vi "Export - Rx Packets.vi"(8 "error in (no error)":errorcluster, 11 "Device Item Ref in":T5 format="%.0x") -> (0 "error out":errorcluster, 3 "Rx Packets":T1 {"Rx Packet Data"."Endianness" items=["big-endian"=0, "little-endian"=2]})   [LabVIEW 2016, in "UDP-Custom-Device System Explorer.lvlib"]
uses:
  UDP-Custom-Device System Explorer.lvlib
  <vilib>/NI Veristand/Custom Device API/Custom Device Item Ref.ctl
  Types/XML - New/ImpExp - Rx Packets Data.ctl
  <vilib>/NI Veristand/Custom Device API/Custom Device Item Info.ctl
  Types/XML - New/ImpExp - Rx Packet Data.ctl
  Shared/Types/Shared - Channel Data Type.ctl
  <vilib>/NI VeriStand/Custom Device API/Custom Device API.lvlib
  Property Accessors/Shared Section Accessors.lvlib
  Shared/UDP-Custom-Device Shared.lvlib
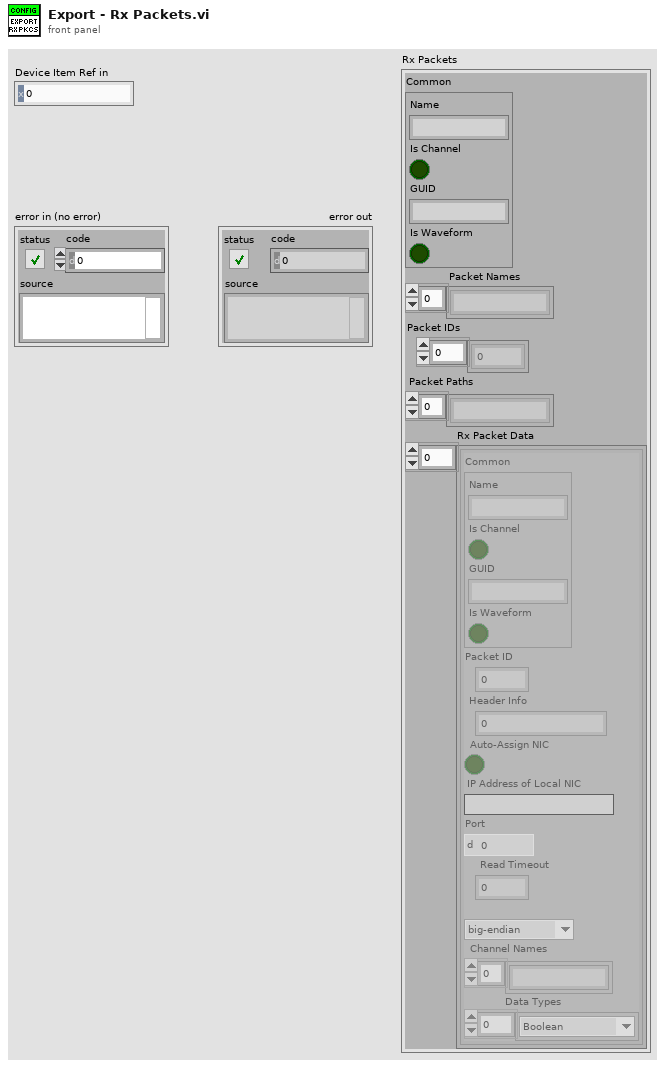
[diagram p1: front panel]
types:
  T1 = typedef "UDP-Custom-Device System Explorer.lvlib/ImpExp - Rx Packets Data.ctl" = cluster{"Common":T2, "Packet Names":string[], "Packet IDs":i32[], "Packet Paths":string[], "Rx Packet Data":T3[]}
  T2 = typedef "Custom Device API.lvlib/Custom Device Item Info.ctl" = cluster{"Name":string, "Is Channel":bool, "GUID":string, "Is Waveform":bool}
  T3 = typedef "UDP-Custom-Device System Explorer.lvlib/ImpExp - Rx Packet Data.ctl" = cluster{"Common":T2, "Packet ID":i32, "Header Info":u32, "Auto-Assign NIC":bool, "IP Address of Local NIC":string, "Port":u16, "Read Timeout":i32, "Endianness":u16, "Channel Names":string[], "Data Types":T4[]}
  T4 = typedef "UDP-Custom-Device Shared.lvlib/Shared - Channel Data Type.ctl" = enum16{"Boolean", "Single", "Double", "I8", "I16", "I32", "I64", "U8", "U16", "U32", "U64"}
  T5 = typedef "Custom Device API.lvlib/Custom Device Item Ref.ctl" = u64
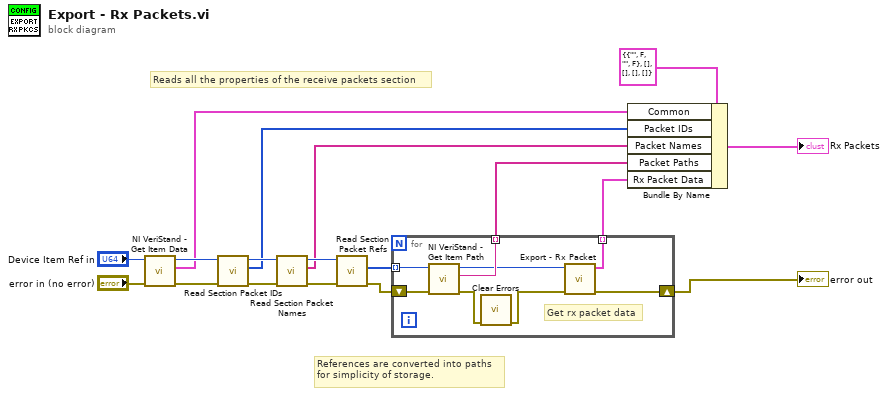
[diagram p0: block diagram]
diagram:
  # "References are converted into paths\nfor simplicity of storage."
  # "Reads all the properties of the receive packets section"
  n1 = call <vilib>:"NI VeriStand - Get Item Data.vi"("error in (no error)"="error in (no error)", "Item Ref in"="Device Item Ref in") -> ("error out"=w13:errorcluster, "Item Info"=w6:T2, "Item Ref out"=w18:T5)  [unwired: 6 in, 1 out]
  n2 = call "Read Section Packet IDs.vi"("error in (no error)"=w13, "Node Ptr"=w18) -> ("error out"=w15:errorcluster, "Packet IDs"=w5:i32[], "Node Ptr out"=w17:T5)  [unwired: 7 in]
  n3 = call "Read Section Packet Names.vi"("error in (no error)"=w15, "Node Ptr"=w17) -> ("error out"=w14:errorcluster, "Packet Names"=w4:string[], "Node Ptr out"=w16:T5)  [unwired: 7 in]
  n4 = call "Read Section Packet Refs.vi"("error in (no error)"=w14, "Node Ptr"=w16) -> ("error out"=w12:errorcluster, "Dependent Node Refs"=w11:T5[])  [unwired: 7 in, 1 out]
  n5 = for {
    shift-right: [w20] -> w8
    shift-left: w12 -> [w26]
    tunnel: w11 -> [w25] mode=indexing
    tunnel: [w24] -> w3 mode=indexing
    tunnel: [w19] -> w1 mode=indexing
    # "Get rx packet data"
    n6 = call <vilib>:"NI VeriStand - Get Item Path.vi"("error in (no error)"=w26, "Item Ref in"=w25) -> ("error out"=w23:errorcluster, "Path"=w24:string, "Item Ref out"=w22:T5)  [unwired: 6 in, 1 out]
    n7 = call <vilib>:"Clear Errors.vi"("error in (no error)"=w23) -> ("error out"=w21:errorcluster)  [unwired: 5 in, 1 out]
    n8 = call "Export - Rx Packet.vi"("error in (no error)"=w21, "Device Item Ref in"=w22) -> ("error out"=w20:errorcluster, "Rx Packet"=w19:T3)  [unwired: 8 in]
  }
  "error out" <- w8
  n9 = Bundle By Name(cluster=T1 {"Common"={"Name"="", "Is Channel"=FALSE, "GUID"="", "Is Waveform"=FALSE}, "Packet Names"=[], "Packet IDs"=[], "Packet Paths"=[], "Rx Packet Data"=[]} ("Rx Packets"), "Common"=w6, "Packet IDs"=w5, "Packet Names"=w4, "Packet Paths"=w3, "Rx Packet Data"=w1) -> (→"Rx Packets":T1)
